vi "PXI-2514.Async.vi"(10 "Parameters":variant, 11 "Process":refnum<class "Process.lvclass">) -> ()   [LabVIEW 2020, in "PXI-2514 Engine.lvlib"]
uses:
  <vilib>/NI/NIVS Inline Async API/_VS Inline Async API/Process/Process.lvclass
  <vilib>/NI/NIVS Inline Async API/_VS Inline Async API/Process/Process.lvclass/Process.ctl
  <vilib>/NI/NIVS Inline Async API/_Data Access Engine/Access Type Classes/Read/Read.lvclass/Read.ctl
  <vilib>/NI/NIVS Inline Async API/_Data Access Engine/Access Type Classes/Write/Write.lvclass/Write.ctl
  <vilib>/NI/NIVS Inline Async API/_Data Access Engine/Data Access Engine/Methods/Read.Data.vi
  <vilib>/NI/NIVS Inline Async API/_VS Inline Async API/Process/Data Member Access/Read Data Access.vi
  <vilib>/NI/NIVS Inline Async API/_VS Inline Async API/Error Handling Process/SubVIs/Error.ConvertArray.vi
  <vilib>/NI/NIVS Inline Async API/_Data Access Engine/Access Type Classes/Read/Read.ProcessData.vi
  <vilib>/NI/NIVS Inline Async API/_Data Access Engine/Access Type Classes/Write/Write.ProcessData.vi
  <vilib>/NI/NIVS Inline Async API/_Data Access Engine/Access Type Classes/Write/Write.Buffer.vi
  <vilib>/NI/NIVS Inline Async API/_Data Access Engine/Access Type Classes/Write/Write.Commit.vi
  <vilib>/NI/NIVS Inline Async API/_Data Access Engine/Data Access Engine/Data Access Engine.lvclass
  PXI-2514 Engine.lvlib
  <vilib>/NI/NIVS Inline Async API/_Data Access Engine/Data Access Engine/Methods/Read.Lookup.vi
  <vilib>/NI/NIVS Inline Async API/_Data Access Engine/Data Access Engine/Methods/Write.Lookup.vi
  <vilib>/NI/NIVS Inline Async API/_Data Access Engine/Data Access Engine/Methods/Write.Data.vi
  Shared/Compiled.Settings.ctl
  Shared/PXI-2514 Shared.lvlib
  <instrlib>/niSwitch/niSwitch.llb/niSwitch Topologies.ctl
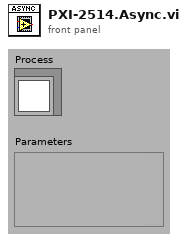
[diagram p1: front panel]
types:
  T1 = typedef "niSwitch Topologies.ctl" = string
  T2 = typedef "PXI-2514 Shared.lvlib/Compiled.Settings.ctl" = cluster{"Name":string, "Async Init Timeout":u16, "Hardware Device Name":string}
  T3 = typedef "Data Access Engine.lvlib/Data Access Engine.lvclass/Write.DVR.ctl" = refnum<data-value>
  T4 = typedef "Data Access Engine.lvlib/Data Access Engine.lvclass/Read.DVR.ctl" = refnum<data-value>
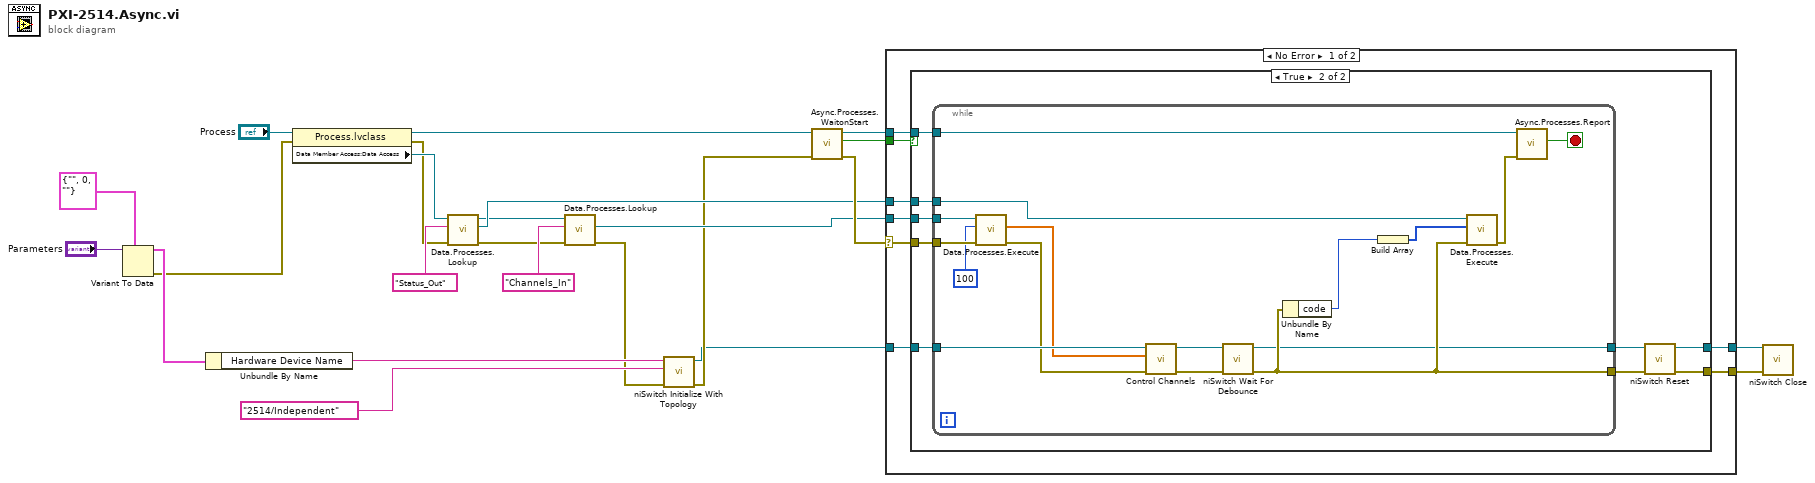
[diagram p0: block diagram]
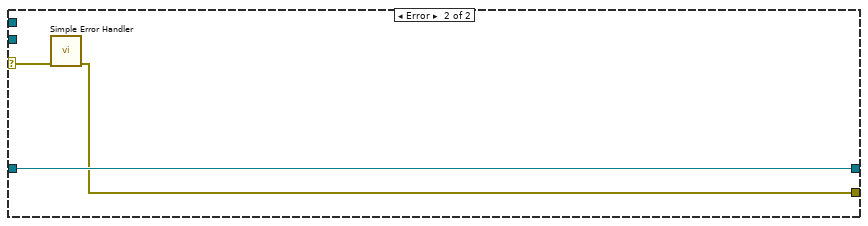
[diagram p3: hidden frame]
diagram:
  n1 = Variant To Data(type=T2 {"Name"="", "Async Init Timeout"=0, "Hardware Device Name"=""} ("Compiled.Settings"), Variant="Parameters") -> (data=w9:T2, error out=w8:errorcluster)  [unwired: 1 in]
  n2 = Unbundle By Name(w9) -> ("Hardware Device Name"=w7:string)
  n3 = property class="Process.lvclass"(reference="Process", error in=w8) -> (reference out=w14:refnum<class "Process.lvclass">, error out=w12:errorcluster, "Data Member Access:Data Access"=w13:refnum<class "Data Access Engine.lvclass">)
  n4 = call-poly <vilib>:"Data.Processes.Lookup.vi"("error in (no error)"=w12, "Name"="Status_Out", "Data Access API in"=w13) -> ("error out"=w18:errorcluster, "Ref"=w17:T3, "Data Access API out"=w16:refnum<class "Data Access Engine.lvclass">)  [unwired: 5 in, 1 out]
  n5 = call-poly <vilib>:"Data.Processes.Lookup.vi"("error in (no error)"=w18, "Name"="Channels_In", "Data Access API in"=w16) -> ("error out"=w5:errorcluster, "Ref"=w20:T4)  [unwired: 5 in, 2 out]
  n6 = call <instrlib>:"niSwitch Initialize With Topology.vi"("error in (no error)"=w5, "topology name"=T1 "2514/Independent", "resource name"=w7) -> ("error out"=w4:errorcluster, "instrument handle out"=w3:refnum<k15>)  [unwired: 7 in]
  n7 = call <vilib>:"Async.Processes.WaitonStart.vi"("error in (no error)"=w4, "Process"=w14) -> ("error out"=w22:errorcluster, "Execute"=w24:bool, "Process out"=w23:refnum<class "Process.lvclass">)  [unwired: 7 in]
  n8 = case shown="No Error" w22 {
    selector: w22 -> [w28 w62]
    tunnel: w24 -> [w32 _]
    tunnel: w23 -> [w31 _]
    tunnel: w17 -> [w30 _]
    tunnel: w20 -> [w29 _]
    tunnel: w3 -> [w27 w61]
    tunnel: [w26 w61] -> w2
    tunnel: [w25 w60] -> w1
    frame No Error {
      n9 = case shown="True" w32 {
        tunnel: w28 -> [w34 w40]
        tunnel: w31 -> [_ w41]
        tunnel: w29 -> [_ w43]
        tunnel: w30 -> [_ w42]
        tunnel: w27 -> [w33 w39]
        tunnel: [w33 w36] -> w26
        tunnel: [w34 w35] -> w25
        frame False {
        }
        frame True {
          n10 = while {
            tunnel: w40 -> [w55]
            tunnel: w41 -> [w59]
            tunnel: w43 -> [w57]
            tunnel: w42 -> [w56]
            tunnel: w39 -> [w52]
            tunnel: [w45] -> w38
            tunnel: [w44] -> w37
            stop <- w58 stop-if-true
            n11 = call-poly <vilib>:"Data.Processes.Execute.vi"("error in (no error)"=w55, "timeout ms"=100, "Ref"=w57) -> ("error out"=w51:errorcluster, "Values"=w50:dbl[])  [unwired: 6 in, 1 out]
            n12 = call "Control Channels.vi"("error in (no error)"=w51, "Array"=w50, "IVI Refnum in"=w52) -> ("error out"=w48:errorcluster, "IVI Refnum out"=w49:refnum<k15>)  [unwired: 7 in]
            n13 = call <instrlib>:"niSwitch Wait For Debounce.vi"("error in (no error)"=w48, "instrument handle"=w49) -> ("error out"=w45:errorcluster, "instrument handle out"=w44:refnum<k15>)  [unwired: 8 in]
            n14 = Unbundle By Name(w45) -> ("code"=w47:i32)
            n15 = Build Array(w47) -> (w46:i32[])
            n16 = call-poly <vilib>:"Data.Processes.Execute.vi"("error in (no error)"=w45, "Values"=w46, "Ref"=w56) -> ("error out"=w53:errorcluster)  [unwired: 8 in]
            n17 = call <vilib>:"Async.Processes.Report.vi"("Error"=w53, "Process in"=w59) -> ("Stop"=w58:bool)  [unwired: 8 in, 1 out]
          }
          n18 = call <instrlib>:"niSwitch Reset.vi"("error in (no error)"=w38, "instrument handle"=w37) -> ("error out"=w35:errorcluster, "instrument handle out"=w36:refnum<k15>)  [unwired: 8 in]
        }
      }
    }
    frame Error {
      n19 = call <vilib>:"Simple Error Handler.vi"("error in (no error)"=w62) -> ("error out"=w60:errorcluster)  [unwired: 4 in, 4 out]
    }
  }
  n20 = call <instrlib>:"niSwitch Close.vi"("error in (no error)"=w1, "instrument handle"=w2) -> ()  [unwired: 9 in, 1 out]
